vi "Build XY Plot Histogram (Core).vi"(6 "Plot Index (-1: last)":i32=-1, 7 "Data Axis (Y: F)":bool, 8 "error in (no error)":errorcluster, 9 "Histogram Options (Default: dialog)":T1={"Bin Size"=nan, "Bin Number"=0, "Bin Option"=enum."Bin Number", "Min Value"=-inf, "Max Value"=inf, "Filter NaN & Infinite Values"=TRUE, "Frequency Plot"=FALSE, "Align Bins"=TRUE, "Bin Location"=enum."Left", "Project Outside Values"=FALSE, "Max Histogram Size"=100000} {"Max Histogram Size" format="%.0e"}, 10 "Mouse Click Coords (default: use Plot Index)":T4={"Horizontal"=2147483647, "Vertical"=2147483647}, 11 "XY Graph":T5) -> (0 "error out":errorcluster, 1 "Message":string, 3 "Data Statistics":dbl[](array[numeric]))   [LabVIEW 2021, in "Histogram Window.lvlib"]
uses:
  Histogram Window.lvlib
  Graphs/XY Graph/XY Graph Refnum.ctl
  <vilib>/Utility/miscctls.llb/LVPoint32TypeDef.ctl
  Linear Histogram Options.ctl
  Histogram Bin Option.ctl
  Histogram Bin Position.ctl
  Graphs/Get Plot at Mouse Click (XY Graph)/Get Plot at Mouse Click [AAC].vi
  Arrays/Arrays.lvlib
  Graphs/Graphs.lvlib
  Graphs/XY Graph/XY Graph Add-Ons.lvlib
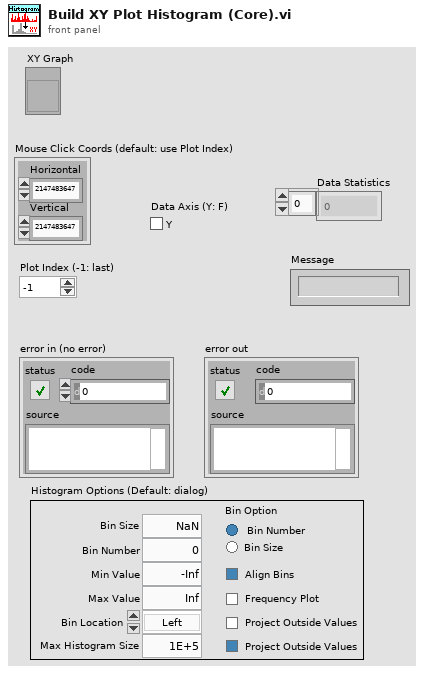
[diagram p1: front panel]
types:
  T1 = typedef "Histogram Window.lvlib/Linear Histogram Options.ctl" = cluster{"Bin Size":dbl, "Bin Number":i32, "Bin Option":T2, "Min Value":dbl, "Max Value":dbl, "Filter NaN & Infinite Values":bool, "Frequency Plot":bool, "Align Bins":bool, "Bin Location":T3, "Project Outside Values":bool, "Max Histogram Size":i32}
  T2 = typedef "Histogram Window.lvlib/Histogram Bin Option.ctl" = enum32{"Bin Number", "Bin Size"}
  T3 = typedef "Histogram Window.lvlib/Histogram Bin Position.ctl" = enum16{"Left", "Center", "Right"}
  T4 = typedef "LVPoint32TypeDef.ctl" = cluster{"Horizontal":i32, "Vertical":i32}
  T5 = typedef "XY Graph Add-Ons.lvlib/XY Graph Refnum.ctl" = refnum<vi>
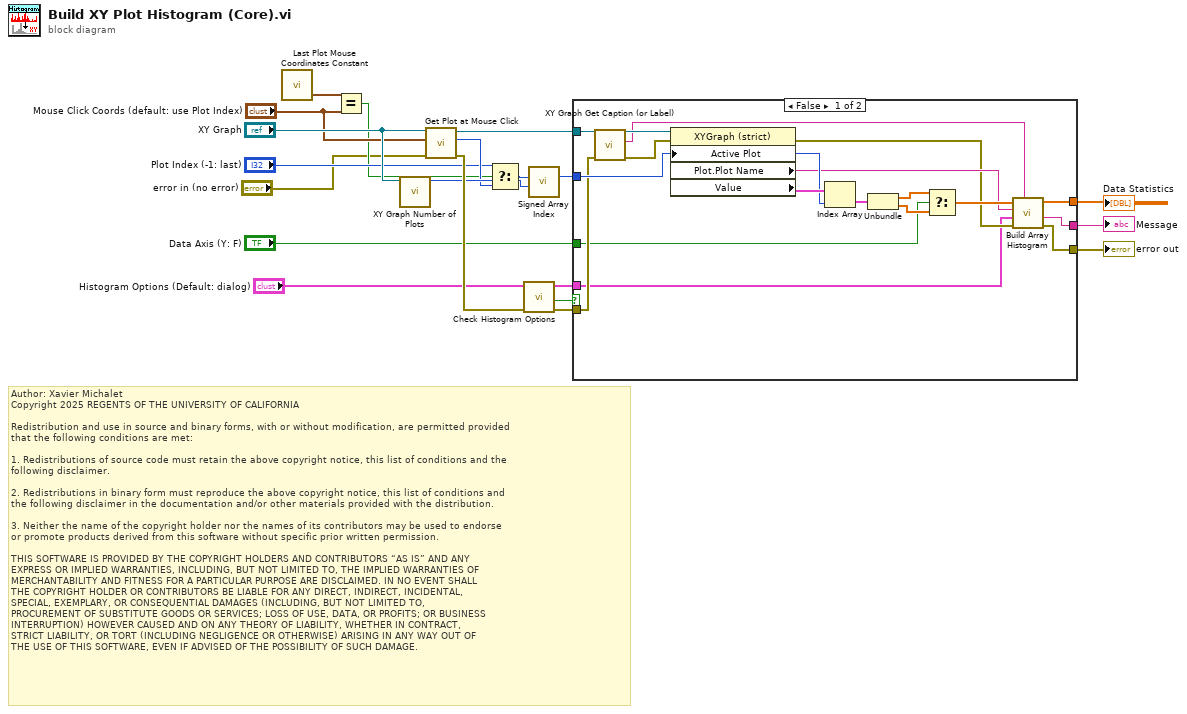
[diagram p0: block diagram]
diagram:
  # "Author: Xavier Michalet\nCopyright 2025 REGENTS OF THE UNIVERSITY OF CALIFORNIA\n\nRedistribution and use in source and binary forms, with or without modification, are permitted provided\nthat the following conditions are met:\n\n1. Redistributions of source code must retain the above copyright notice, this list of conditions and the\nfollowing disclaimer.\n\n2. Redistributions in binary form must reproduce the above copyright notice, this list of conditions and\nthe following disclaimer in the documentation and/or other materials provided with the distribution.\n\n3. Neither the name of the copyright holder nor the names of its contributors may be used to endorse \nor promote products derived from this software without specific prior written permission.\n\nTHIS SOFTWARE IS PROVIDED BY THE COPYRIGHT HOLDERS AND CONTRIBUTORS “AS IS” AND ANY \nEXPRESS OR IMPLIED WARRANTIES, INCLUDING, BUT NOT LIMITED TO, THE IMPLIED WARRANTIES OF\nMERCHANTABILITY AND FITNESS FOR A PARTICULAR PURPOSE ARE DISCLAIMED. IN NO EVENT SHALL\nTHE COPYRIGHT HOLDER OR CONTRIBUTORS BE LIABLE FOR ANY DIRECT, INDIRECT, INCIDENTAL, \nSPECIAL, EXEMPLARY, OR CONSEQUENTIAL DAMAGES (INCLUDING, BUT NOT LIMITED TO, \nPROCUREMENT OF SUBSTITUTE GOODS OR SERVICES; LOSS OF USE, DATA, OR PROFITS; OR BUSINESS\nINTERRUPTION) HOWEVER CAUSED AND ON ANY THEORY OF LIABILITY, WHETHER IN CONTRACT, \nSTRICT LIABILITY, OR TORT (INCLUDING NEGLIGENCE OR OTHERWISE) ARISING IN ANY WAY OUT OF\nTHE USE OF THIS SOFTWARE, EVEN IF ADVISED OF THE POSSIBILITY OF SUCH DAMAGE."
  n1 = call "Last Plot Mouse Coordinates Constant.vi"() -> ("Selected Plots Mouse Coordinates Equivalent"=w6:T4)
  n2 = Equal?(x=w6, y="Mouse Click Coords (default: use Plot Index)") -> (x = y?=w4:bool)
  n3 = call "XY Graph Number of Plots.vi"("XYGraph in"="XY Graph") -> ("# Plots"=w18:i32)  [unwired: 9 in, 1 out]
  n4 = call-poly "Get Plot at Mouse Click.vi"("error in (no error)"="error in (no error)", "Mouse Click Coordinates"="Mouse Click Coords (default: use Plot Index)", "XYGraph Ref"="XY Graph") -> ("error out"=w19:errorcluster, "Plot at Coordinates"=w14:i32, "XYGraph Ref"=w11:T5)  [unwired: 2 in, 4 out]
  n5 = Select(t="Plot Index (-1: last)", s=w4, f=w14) -> (s? t:f=w16:i32)
  n6 = call "Check Histogram Options.vi"("error in (no error)"=w19, "Histogram Options in"="Histogram Options (Default: dialog)") -> ("error out"=w8:errorcluster, "Cancelled?"=w1:bool, "Histogram Options out"=w7:T1)  [unwired: 7 in]
  n7 = call "Signed Array Index.vi"("Array Size"=w18, "Array Index in"=w16) -> ("Array Index out"=w17:i32)  [unwired: 9 in]
  n8 = case shown="False" w1 {
    tunnel: w11 -> [w29 _]
    tunnel: [w32 w39] -> w20
    tunnel: w17 -> [w36 _]
    tunnel: w8 -> [w26 w39]
    tunnel: [w22 _] -> w12
    tunnel: "Data Axis (Y: F)" -> [w23 _]
    tunnel: [w21 _] -> w9
    tunnel: w7 -> [w24 _]
    frame False {
      n9 = call "XY Graph Get Caption (or Label).vi"("error in (no error)"=w26, "XY Graph in"=w29) -> ("error out"=w27:errorcluster, "Caption (or Label) Text"=w25:string, "XY Graph out"=w28:T5)  [unwired: 7 in]
      n10 = property class="XYGraph (strict)"(reference=w28, error in=w27, "Active Plot"=w36) -> (error out=w30:errorcluster, "Plot.Plot Name"=w31:string, "Value"=w38:cluster{"X Array":dbl[], "Y Array":dbl[]}[])  [unwired: 1 out]
      n11 = Index Array(array=w38, index=w36) -> (element=w37:cluster{"X Array":dbl[], "Y Array":dbl[]})
      n12 = Unbundle(w37) -> ("X Array"=w35:dbl[], "Y Array"=w34:dbl[])
      n13 = Select(t=w35, s=w23, f=w34) -> (s? t:f=w33:dbl[])
      n14 = call "Build Array Histogram.vi"("Graph Caption (or Label) Text"=w25, "error in (no error)"=w30, "Histogram Options"=w24, "Plot/Dataset Name"=w31, "Array"=w33) -> ("error out"=w32:errorcluster, "Message"=w21:string, "Data Statistics"=w22:dbl[])  [unwired: 4 in]
    }
    frame True {
    }
  }
  "error out" <- w20
  "Data Statistics" <- w12
  "Message" <- w9
